vi "Do.vi"(8 "error in (no error)":errorcluster, 10 "Actor in":refnum<class "Actor.lvclass">, 11 "Add Customer Msg":refnum<class "Add Customer Msg.lvclass">) -> (0 "error out":errorcluster, 2 "Actor out":refnum<class "Actor.lvclass">)   [LabVIEW 2023, in "Coffee Shop.lvlib" / "Add Customer Msg.lvclass"]
doc: "This VI delivers the message to the actor by calling the appropriate method(s) on the actor."
uses:
  Add Customer Msg.lvclass
  <vilib>/ActorFramework/Actor/Actor.lvclass
  Coffee Shop/Coffee Shop.lvclass
  c:/dev/_r/4/eng/lv-core/lvpostprocessingd/lv_mc_x86_64/dist_i386/vi.lib/ActorFramework/Actor/Actor.lvclass
  Coffee Shop/Entity Types.ctl
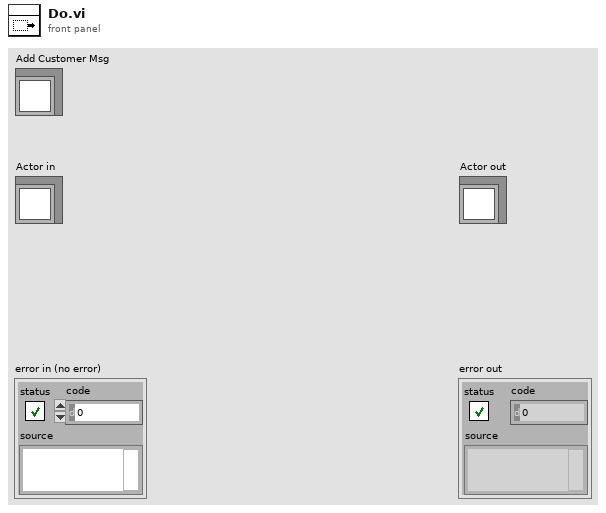
[diagram p1: front panel]
types:
  T1 = typedef "Coffee Shop.lvlib/Coffee Shop.lvclass/Entity Types.ctl" = enum16{"Customer", "Cashier", "Barista"}
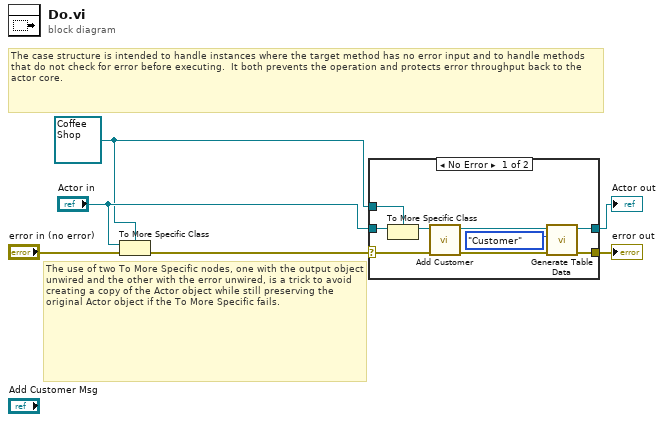
[diagram p0: block diagram]
diagram:
  w1 = refnum<class "Coffee Shop.lvclass"> refnum ("Actor in")
  # "The use of two To More Specific nodes, one with the output object unwired and the other with the error unwired, is a trick to avoid creating a copy of the Actor object while still preserving the original Actor object if the To More Specific fails."
  # "The case structure is intended to handle instances where the target method has no error input and to handle methods that do not check for error before executing.  It both prevents the operation and protects error throughput back to the actor core."
  n1 = To More Specific Class(target class=w1, reference="Actor in", error in="error in (no error)") -> (error out=w5:errorcluster)  [unwired: 1 out]
  n2 = case shown="No Error" w5 {
    selector: w5 -> [w15 w17]
    tunnel: [w10 w17] -> w4
    tunnel: [w11 w16] -> w3
    tunnel: "Actor in" -> [w14 w16]
    tunnel: w1 -> [w13 _]
    frame No Error {
      n3 = To More Specific Class(target class=w13, reference=w14) -> (specific class reference=w12:refnum<class "Coffee Shop.lvclass">)  [unwired: 1 in, 1 out]
      n4 = call-dynamic "Add Customer.vi"("error in (no error)"=w15, "Coffee Shop in"=w12) -> ("error out"=w8:errorcluster, "Coffee Shop out"=w9:refnum<class "Coffee Shop.lvclass">)  [unwired: 8 in]
      n5 = call-dynamic "Generate Table Data.vi"("error in (no error)"=w8, "Entity Type"=Entity_Types."Customer", "Coffee Shop in"=w9) -> ("error out"=w10:errorcluster, "Coffee Shop out"=w11:refnum<class "Coffee Shop.lvclass">)  [unwired: 7 in]
    }
    frame Error {
      # "If type check fails, pass the original object out again."
    }
  }
  "error out" <- w4
  "Actor out" <- w3
